vi "File.String Array to CSV.vi"(8 "Error In":errorcluster, 10 "2D Str":string[][](array[string]), 11 "FilePath":path) -> (0 "Error Out":errorcluster, 3 "FilePath Out":path)   [LabVIEW 2024]
uses:
  <vilib>/KATE/Files/File Utils.lvlib
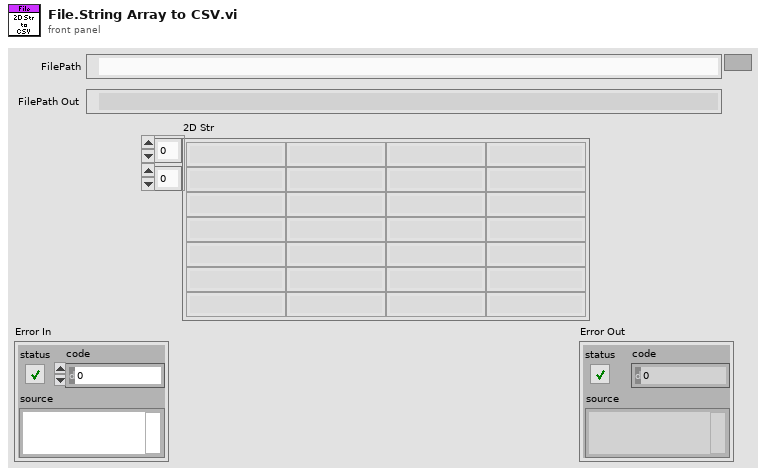
[diagram p1: front panel]
types:
  T1 = enum16{"open", "replace", "create", "open or create", "replace or create", "replace or create with confirmation"}
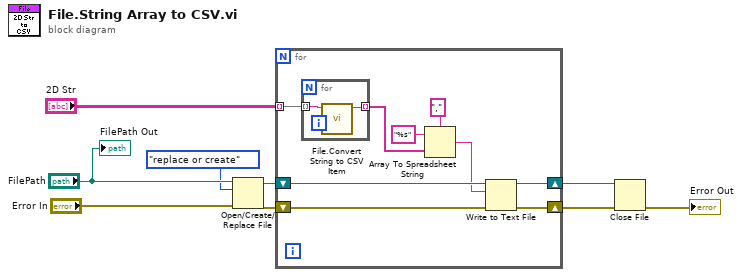
[diagram p0: block diagram]
diagram:
  n1 = Open/Create/Replace File(file path (use dialog)="FilePath", error in="Error In", operation (0:open)=T1."replace or create") -> (refnum out=w7:refnum<file>, error out=w6:errorcluster)  [unwired: 3 in, 1 out]
  n2 = for {
    shift-right: [w17] -> w9
    shift-left: w7 -> [w15]
    shift-right: [w16] -> w8
    shift-left: w6 -> [w13]
    tunnel: "2D Str" -> [w12] mode=indexing
    n3 = for {
      tunnel: w12 -> [w19] mode=indexing
      tunnel: [w20] -> w11 mode=indexing
      n4 = call <vilib>:"File.Convert String to CSV Item.vi"("String"=w19) -> ("String Out"=w20:string)  [unwired: 10 in]
    }
    n5 = Array To Spreadsheet String(delimiter (Tab)=",", array=w11, 3:"%s" ("format string")) -> (spreadsheet string=w14:string)
    n6 = Write to Text File(file (use dialog)=w15, text=w14, error in=w13) -> (refnum out=w17:refnum<file>, error out=w16:errorcluster)  [unwired: 1 in, 1 out]
  }
  n7 = Close File(refnum=w9, error in=w8) -> (error out=→"Error Out":errorcluster)  [unwired: 1 out]
  "FilePath Out" <- "FilePath"
